vi "ExtractControlRefs.vi"(7 "Indicators":bool, 8 "error in (no error)":errorcluster, 10 "ShowAllControls?":bool, 11 "VI in":refnum<vi>) -> (0 "error out":errorcluster, 3 "Controls":T1[](array[typedef]))   [LabVIEW 2017, in "ContextHelpEditor.lvlib"]
uses:
  ContextHelpEditor.lvlib
  ControlRef--cluster.ctl
  <vilib>/picture/picture.llb/imagedata.ctl
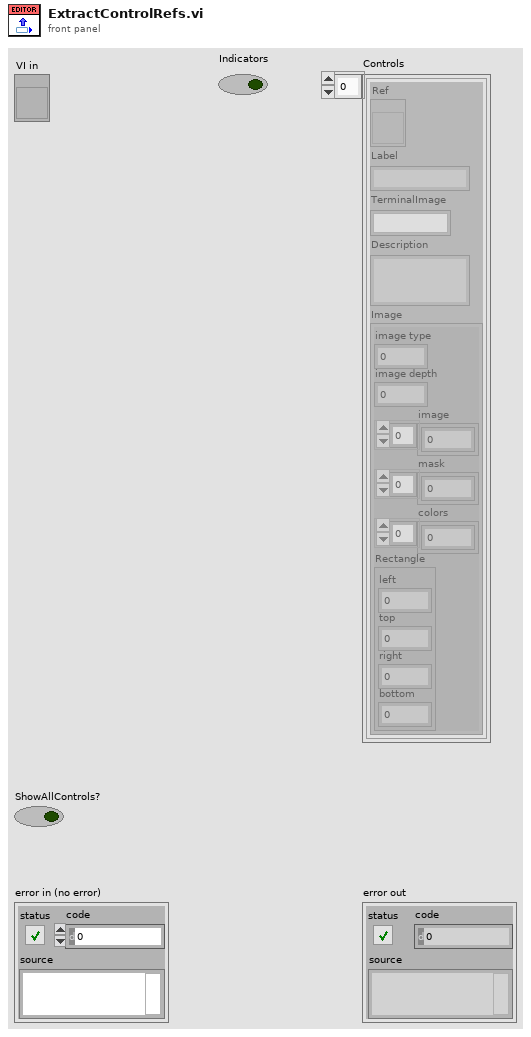
[diagram p1: front panel]
types:
  T1 = typedef "ContextHelpEditor.lvlib/ControlRef--cluster.ctl" = cluster{"Ref":refnum<vi>, "Label":string, "TerminalImage":picture, "Description":string, "Image":T2}
  T2 = typedef "imagedata.ctl" = cluster{"image type":i32, "image depth":i32, "image":u8[], "mask":u8[], "colors":u32[], "Rectangle":cluster{"left":i16, "top":i16, "right":i16, "bottom":i16}}
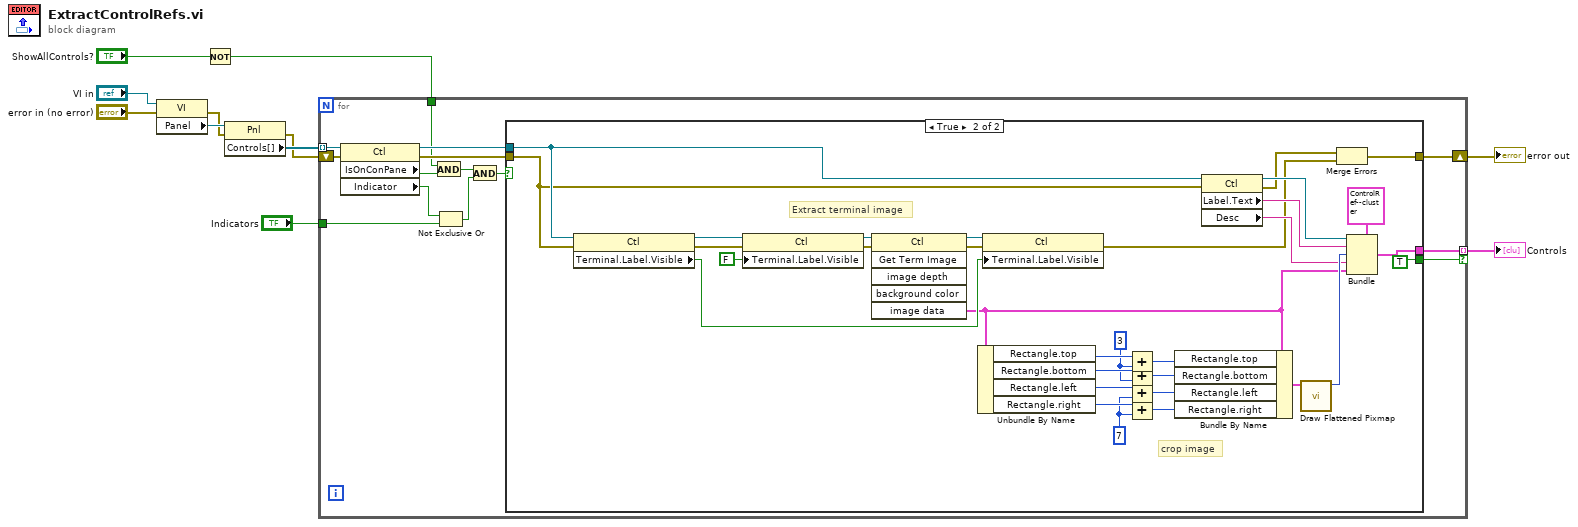
[diagram p0: block diagram]
diagram:
  n1 = property class="VI"(reference="VI in", error in="error in (no error)") -> (error out=w7:errorcluster, "Panel"=w10:refnum<vi>)  [unwired: 1 out]
  n2 = Not(x="ShowAllControls?") -> (.not. x?=w1:bool)
  n3 = property class="Pnl"(reference=w10, error in=w7) -> (error out=w6:errorcluster, "Controls[]"=w11:refnum<vi>[])  [unwired: 1 out]
  n4 = for {
    tunnel: w11 -> [w25] mode=indexing
    tunnel: [w21] -> w5 mode=indexing if=w14
    shift-right: [w19] -> w4
    shift-left: w6 -> [w22]
    tunnel: "Indicators" -> [w16]
    tunnel: w1 -> [w12]
    n5 = property class="Ctl"(reference=w25, error in=w22) -> (reference out=w24:refnum<vi>, error out=w20:errorcluster, "IsOnConPane"=w23:bool, "Indicator"=w17:bool)
    n6 = And(x=w12, y=w23) -> (x .and. y?=w13:bool)
    n7 = Not Exclusive Or(1:w16, 2:w17) -> (0:w15:bool)
    n8 = And(x=w13, y=w15) -> (x .and. y?=w18:bool)
    n9 = case shown="True" w18 {
      tunnel: w24 -> [_ w41]
      tunnel: [_ w53] -> w21
      tunnel: w20 -> [w26 w40]
      tunnel: [w26 w50] -> w19
      tunnel: [_ TRUE] -> w14
      frame False {
      }
      frame True {
        w30 = i16 7 ("y")
        w35 = i16 3 ("y")
        # "crop image"
        # "Extract terminal image"
        n10 = property class="Ctl"(reference=w41, error in=w40) -> (reference out=w42:refnum<vi>, error out=w43:errorcluster, "Terminal.Label.Visible"=w39:bool)
        n11 = property class="Ctl"(reference=w42, error in=w43, "Terminal.Label.Visible"=FALSE) -> (reference out=w47:refnum<vi>, error out=w48:errorcluster)
        n12 = invoke class="Ctl" method="Get Term Image"(reference=w47, error in=w48) -> (reference out=w44:refnum<vi>, error out=w52:errorcluster, "image data"=w27:T2)  [unwired: 4 in, 3 out]
        n13 = Unbundle By Name(w27) -> ("Rectangle.top"=w38:i16, "Rectangle.bottom"=w36:i16, "Rectangle.left"=w34:i16, "Rectangle.right"=w33:i16)
        n14 = property class="Ctl"(reference=w44, error in=w52, "Terminal.Label.Visible"=w39) -> (error out=w45:errorcluster)  [unwired: 1 out]
        n15 = Add(x=w38, y=w35) -> (x+y=w37:i16)
        n16 = Add(x=w36, y=w35) -> (x+y=w29:i16)
        n17 = Add(x=w34, y=w30) -> (x+y=w32:i16)
        n18 = Add(x=w33, y=w30) -> (x+y=w31:i16)
        n19 = Bundle By Name(cluster=w27, "Rectangle.top"=w37, "Rectangle.bottom"=w29, "Rectangle.left"=w32, "Rectangle.right"=w31) -> (w28:T2)
        n20 = property class="Ctl"(reference=w41, error in=w40) -> (reference out=w55:refnum<vi>, error out=w51:errorcluster, "Label.Text"=w56:string, "Desc"=w54:string)
        n21 = call <vilib>:"Draw Flattened Pixmap.vi"("image data"=w28) -> ("new picture"=w57:picture)  [unwired: 8 in]
        n22 = Merge Errors(w51, w45) -> (w50:errorcluster)
        n23 = Bundle(cluster=T1 {"Ref"=refnum, "Label"="", "TerminalImage"=bytes[0], "Description"="", "Image"={"image type"=0, "image depth"=0, "image"=[], "mask"=[], "colors"=[], "Rectangle"={"left"=0, "top"=0, "right"=0, "bottom"=0}}} ("ControlRef"), "Ref"=w55, "Label"=w56, "TerminalImage"=w57, "Description"=w54, "Image"=w27) -> (w53:T1)
      }
    }
  }
  "error out" <- w4
  "Controls" <- w5
